vi "PWM_Conversion (SubVI).vi"(8 "Min Linear Velocity (ft/s)":dbl=-2.0 format="%#_13g", 9 "Max Linear Velocity (ft/s)":dbl=2.0 format="%#_13g", 10 "PWM Frequency":dbl=333.33 format="%#_13g", 11 "Linear Velocity Input (ft/s)":dbl) -> (3 "PWM Signal Output":dbl)   [LabVIEW 2015]
panel:
  # "Input"
  # "Output"
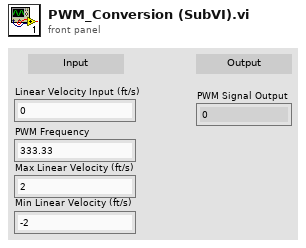
[diagram p1: front panel]
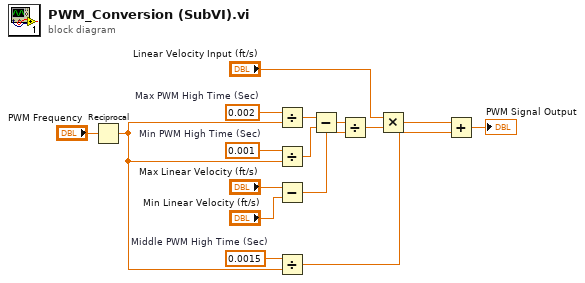
[diagram p0: block diagram]
diagram:
  w2 = 0.0015  # Middle PWM High Time (Sec)
  w7 = 0.001  # Min PWM High Time (Sec)
  w8 = 0.002  # Max PWM High Time (Sec)
  n1 = Reciprocal(x="PWM Frequency") -> (1/x=w3:dbl)
  n2 = Divide(x=w8, y=w3) -> (x/y=w10:dbl)
  n3 = Divide(x=w7, y=w3) -> (x/y=w9:dbl)
  n4 = Subtract(x="Max Linear Velocity (ft/s)", y="Min Linear Velocity (ft/s)") -> (x-y=w6:dbl)
  n5 = Divide(x=w2, y=w3) -> (x/y=w1:dbl)
  n6 = Subtract(x=w10, y=w9) -> (x-y=w4:dbl)
  n7 = Divide(x=w4, y=w6) -> (x/y=w5:dbl)
  n8 = Multiply(x="Linear Velocity Input (ft/s)", y=w5) -> (x*y=w14:dbl)
  n9 = Add(x=w14, y=w1) -> (x+y=→"PWM Signal Output":dbl)
